vi "LED Stand-alone.vi"   [LabVIEW 2015]
uses:
  <vilib>/FPGAPlugInAG/myRIO-1900/niLvFpga_Open_myRIO-1900.vi
  <vilib>/rvi/interface/common/dynamic/niFpgaDynamicAddResources.vi
  <vilib>/FPGAPlugInAG/Dynamic/niLvFpga_Run_Dynamic.vi
  <vilib>/FPGAPlugInAG/Dynamic/niLvFpga_Close_Dynamic.vi
  <vilib>/rvi/interface/nirviOpenFPGA/nirviOpenFPGA.xnode
  FPGA Bitfiles/PDMSMain_FPGATarget-Wi-Fi_Express2_Jo8xc+hAvHc.lvbitx
  FPGA/Express.vi
  <vilib>/rvi/interface/nirviMethod/nirviMethod.xnode
  <vilib>/rvi/interface/nirviCloseFPGA/nirviCloseFPGA.xnode
  FPGA Ref Out.ctl
types:
  T1 = cluster{"LED 3":enum16{"Brightness", "Bool"}, "BOOL":bool, "Brightness":u32}
  T2 = cluster{"LED 2":enum16{"Brightness", "Bool"}, "BOOL":bool, "Brightness":u32}
  T3 = cluster{"LED 0":enum16{"Brightness", "Bool"}, "BOOL":bool, "Brightness":u32}
  T4 = cluster{"LED 1":enum16{"Brightness", "Bool"}, "BOOL":bool, "Brightness":u32}
  T5 = typedef "FPGA Ref Out.ctl" = refnum<k20>
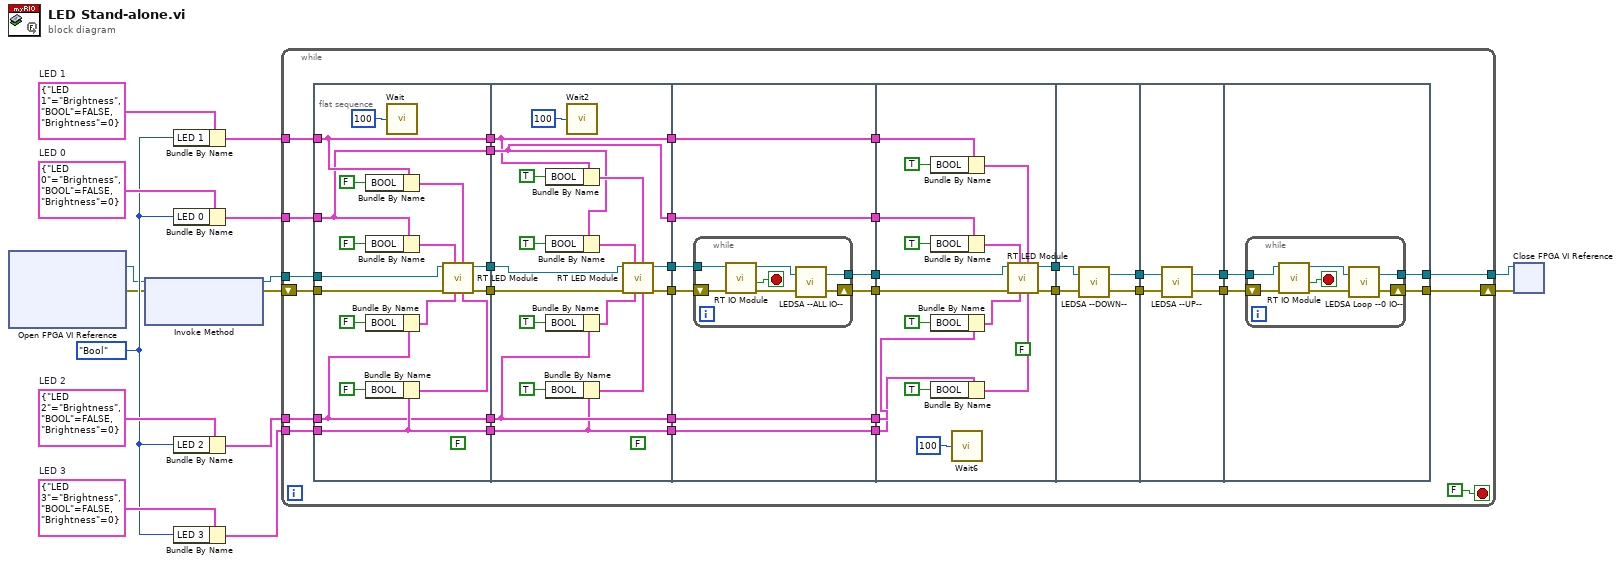
[diagram p0: block diagram]
diagram:
  w11 = enum16{"Brightness", "Bool"}."Bool" ("LED")
  w12 = T1 {"LED 3"=enum."Brightness", "BOOL"=FALSE, "Brightness"=0}  # LED 3
  w13 = T2 {"LED 2"=enum."Brightness", "BOOL"=FALSE, "Brightness"=0}  # LED 2
  w14 = T3 {"LED 0"=enum."Brightness", "BOOL"=FALSE, "Brightness"=0}  # LED 0
  w15 = T4 {"LED 1"=enum."Brightness", "BOOL"=FALSE, "Brightness"=0}  # LED 1
  n1 = xnode "Open FPGA VI Reference"() -> ("FPGA VI Reference Out"=w4:refnum<k20>, "error out"=w3:errorcluster)  [unwired: 2 in]
  n2 = xnode "Invoke Method"("FPGA VI Reference In"=w4, "error in"=w3) -> ("FPGA VI Reference Out"=w2:refnum<k20>, "error out"=w1:errorcluster)  [unwired: 1 in]
  n3 = Bundle By Name(cluster=w15, "LED 1"=w11) -> (w10:T4)
  n4 = Bundle By Name(cluster=w14, "LED 0"=w11) -> (w7:T3)
  n5 = Bundle By Name(cluster=w13, "LED 2"=w11) -> (w8:T2)
  n6 = Bundle By Name(cluster=w12, "LED 3"=w11) -> (w9:T1)
  n7 = while {
    shift-right: [w45] -> w5
    shift-left: w1 -> [w44]
    tunnel: w10 -> [w27]
    tunnel: w9 -> [w26]
    tunnel: w8 -> [w25]
    tunnel: w7 -> [w24]
    tunnel: [w17] -> w6
    tunnel: w2 -> [w16]
    stop <- FALSE stop-if-true
    n8 = flat-sequence {
      tunnel: w44 -> [w65]
      tunnel: [w64] -> w47
      tunnel: [w55] -> w39
      tunnel: [w58] -> w36
      tunnel: [w56] -> w33
      tunnel: [w57] -> w28
      tunnel: w27 -> [w58]
      tunnel: w26 -> [w57]
      tunnel: w25 -> [w56]
      tunnel: w24 -> [w55]
      tunnel: [w50] -> w23
      tunnel: w16 -> [w49]
      tunnel: w47 -> [w82]
      tunnel: [w80] -> w40
      tunnel: w39 -> [w75]
      tunnel: [w75] -> w37
      tunnel: w36 -> [w74]
      tunnel: [w74] -> w34
      tunnel: w33 -> [w73]
      tunnel: [w73] -> w31
      tunnel: [w72] -> w30
      tunnel: w28 -> [w72]
      tunnel: w23 -> [w67]
      tunnel: [w66] -> w22
      tunnel: [w90] -> w41
      tunnel: w40 -> [w89]
      tunnel: [w88] -> w38
      tunnel: w37 -> [w88]
      tunnel: [w87] -> w35
      tunnel: w34 -> [w87]
      tunnel: [w86] -> w32
      tunnel: w31 -> [w86]
      tunnel: w30 -> [w85]
      tunnel: [w85] -> w29
      tunnel: w22 -> [w84]
      tunnel: [w83] -> w21
      tunnel: [w113] -> w46
      tunnel: w41 -> [w112]
      tunnel: w38 -> [w107]
      tunnel: w35 -> [w106]
      tunnel: w32 -> [w105]
      tunnel: w29 -> [w104]
      tunnel: w21 -> [w99]
      tunnel: [w98] -> w20
      tunnel: w46 -> [w118]
      tunnel: [w117] -> w42
      tunnel: w20 -> [w116]
      tunnel: [w115] -> w19
      tunnel: [w121] -> w43
      tunnel: w42 -> [w122]
      tunnel: w19 -> [w120]
      tunnel: [w119] -> w18
      tunnel: [w126] -> w45
      tunnel: w43 -> [w123]
      tunnel: w18 -> [w125]
      tunnel: [w124] -> w17
      frame #0 {
        (unwired) FALSE ("Stop Button")
        n9 = Bundle By Name(cluster=w58, "BOOL"=FALSE ("LED 2")) -> (w59:T4)
        n10 = Bundle By Name(cluster=w55, "BOOL"=FALSE ("LED 0")) -> (w60:T3)
        n11 = Bundle By Name(cluster=w56, "BOOL"=FALSE ("LED 3")) -> (w61:T2)
        n12 = Bundle By Name(cluster=w57, "BOOL"=FALSE ("LED 1")) -> (w62:T1)
        n13 = call "Wait"("Count(mSec)"=u32 100) -> ()  [unwired: 1 out]
        n14 = call "RT LED Module.vi"("LED 3"=w62, "LED 1"=w59, "LED 2"=w61, "LED 0"=w60, "error in"=w65, "FPGA VI Reference In"=w49) -> ("error out"=w64:errorcluster, "FPGA VI Reference Out"=w50:refnum<k20>)  [unwired: 4 in]
      }
      frame #1 {
        (unwired) FALSE ("Stop Button")
        n15 = Bundle By Name(cluster=w74, "BOOL"=TRUE ("LED 2")) -> (w77:T4)
        n16 = Bundle By Name(cluster=w75, "BOOL"=TRUE ("LED 1")) -> (w76:T3)
        n17 = Bundle By Name(cluster=w73, "BOOL"=TRUE ("LED 3")) -> (w78:T2)
        n18 = Bundle By Name(cluster=w72, "BOOL"=TRUE ("LED 0")) -> (w79:T1)
        n19 = call "Wait2"("Count(mSec)"=u32 100) -> ()  [unwired: 1 out]
        n20 = call "RT LED Module.vi"("LED 3"=w79, "LED 1"=w77, "LED 2"=w78, "LED 0"=w76, "error in"=w82, "FPGA VI Reference In"=w67) -> ("error out"=w80:errorcluster, "FPGA VI Reference Out"=w66:refnum<k20>)  [unwired: 4 in]
      }
      frame #2 {
        n21 = while {
          tunnel: w84 -> [w93]
          tunnel: [w96] -> w83
          shift-right: [w97] -> w90
          shift-left: w89 -> [w92]
          stop <- w91 stop-if-true
          n22 = call "RT IO Module.vi"("FPGA VI Reference In"=w93, "Error In"=w92) -> ("FPGA VI Reference Out"=w95:refnum<k20>, "Button"=w91:bool, "Error Out"=w94:errorcluster)  [unwired: 2 in, 4 out]
          n23 = call "LEDSA --ALL IO--.vi"("Error In 2"=w94, "FPGA VI Reference In"=w95) -> ("Error Out 2"=w97:errorcluster, "FPGA VI Reference Out"=w96:T5)
        }
      }
      frame #3 {
        (unwired) FALSE ("Stop Button")
        n24 = Bundle By Name(cluster=w106, "BOOL"=TRUE ("LED 1")) -> (w109:T4)
        n25 = Bundle By Name(cluster=w107, "BOOL"=TRUE ("LED 2")) -> (w108:T3)
        n26 = Bundle By Name(cluster=w105, "BOOL"=TRUE ("LED 3")) -> (w110:T2)
        n27 = Bundle By Name(cluster=w104, "BOOL"=TRUE ("LED 0")) -> (w111:T1)
        n28 = call "Wait6"("Count(mSec)"=u32 100) -> ()  [unwired: 1 out]
        n29 = call "RT LED Module.vi"("LED 3"=w111, "LED 1"=w109, "LED 2"=w110, "LED 0"=w108, "error in"=w112, "FPGA VI Reference In"=w99) -> ("error out"=w113:errorcluster, "FPGA VI Reference Out"=w98:T5)  [unwired: 4 in]
      }
      frame #4 {
        n30 = call "LEDSA --DOWN--.vi"("Error In"=w118, "FPGA VI Reference In"=w116) -> ("Error Out"=w117:errorcluster, "FPGA VI Reference Out"=w115:T5)
      }
      frame #5 {
        n31 = call "LEDSA --UP--.vi"("Error In"=w122, "FPGA VI Reference In"=w120) -> ("Error Out"=w121:errorcluster, "FPGA VI Reference Out"=w119:T5)
      }
      frame #6 {
        n32 = while {
          tunnel: w125 -> [w129]
          tunnel: [w132] -> w124
          shift-right: [w133] -> w126
          shift-left: w123 -> [w127]
          stop <- w128 stop-if-true
          n33 = call "RT IO Module.vi"("FPGA VI Reference In"=w129, "Error In"=w127) -> ("FPGA VI Reference Out"=w131:T5, "Button"=w128:bool, "Error Out"=w130:errorcluster)  [unwired: 2 in, 4 out]
          n34 = call "LEDSA Loop --0 IO--.vi"("Error In"=w130, "FPGA VI Reference In"=w131) -> ("Error Out"=w133:errorcluster, "FPGA VI Reference Out"=w132:T5)
        }
      }
    }
  }
  n35 = xnode "Close FPGA VI Reference"("FPGA VI Reference In"=w6, "error in"=w5) -> ()  [unwired: 1 out]
